vi "MSScript_Calc_ArrayLen.vi"(6 "Value Error?":bool[](array[boolean]), 8 "ArrayVariable in":ext[](array[numeric]), 9 "Param Items":i32) -> (0 "ArrayVariable out":ext[](array[numeric]), 2 "CmdError?":bool)   [LabVIEW 2018, in "MSScript.lvclass"]
uses:
  MSScript.lvclass
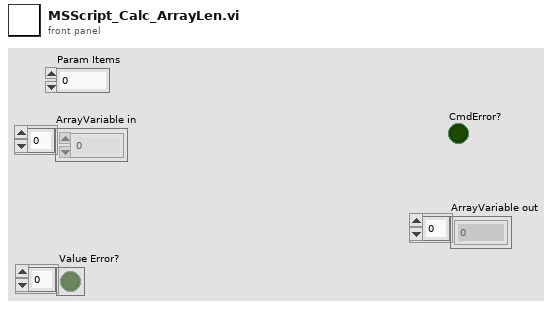
[diagram p1: front panel]
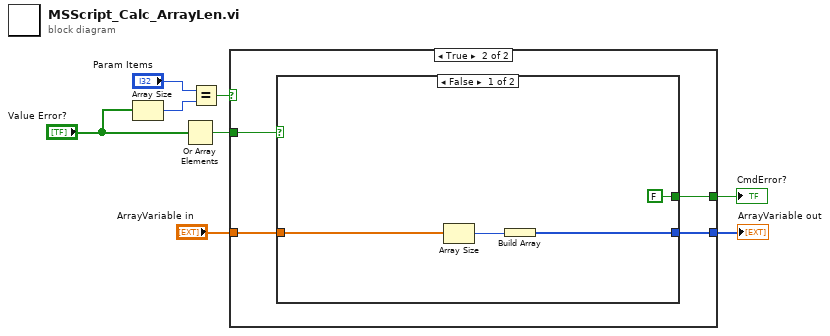
[diagram p0: block diagram]
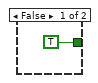
[diagram p2: hidden frame]
diagram:
  n1 = Array Size(array="Value Error?") -> (size(s)=w5:i32)
  n2 = Or Array Elements(Boolean array="Value Error?") -> (logical OR=w7:bool)
  n3 = Equal?(x="Param Items", y=w5) -> (x = y?=w3:bool)
  n4 = case shown="True" w3 {
    tunnel: [TRUE w10] -> w2
    tunnel: w7 -> [_ w13]
    tunnel: [_ w11] -> w8
    tunnel: "ArrayVariable in" -> [_ w12]
    frame False {
    }
    frame True {
      n5 = case shown="False" w13 {
        tunnel: w12 -> [w17 _]
        tunnel: [w14 _] -> w11
        tunnel: [FALSE ("Value Error?") _] -> w10
        frame False {
          n6 = Array Size(array=w17) -> (size(s)=w15:i32)
          n7 = Build Array(w15) -> (w14:i32[])
        }
        frame True {
        }
      }
    }
  }
  "ArrayVariable out" <- w8
  "CmdError?" <- w2
